vi "Read Voltage.vi"(8 "error in)":errorcluster, 11 "Voltmeter CFG in":refnum<class "Voltmeter CFG.lvclass">) -> (0 "error out":errorcluster, 2 "Voltage":dbl format="%#_g V", 3 "Voltmeter CFG out":refnum<class "Voltmeter CFG.lvclass">)   [LabVIEW 2023, in "RIGOL DS1054Z.lvlib" / "Voltmeter CFG.lvclass"]
uses:
  Voltmeter CFG.lvclass
  <vilib>/Analysis/baseanly.llb/Mean (DBL).vi
  Voltmeter CFG.lvclass/Voltmeter CFG.ctl
  <vilib>/Analysis/NI_AALBase.lvlib
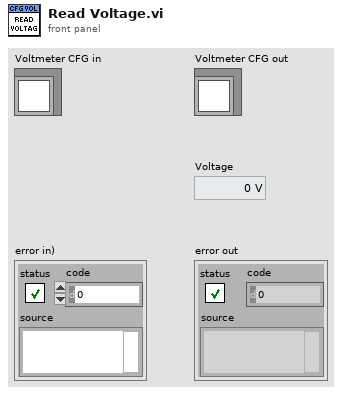
[diagram p1: front panel]
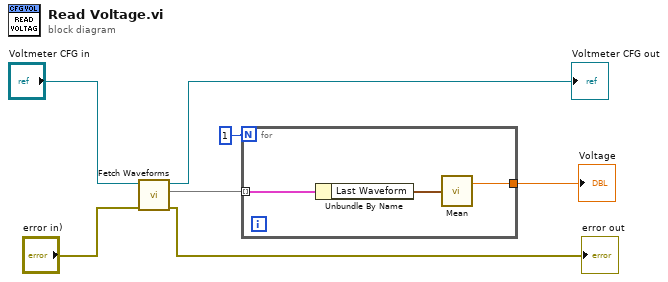
[diagram p0: block diagram]
diagram:
  n1 = call-dynamic "Fetch Waveforms.vi"("error in"="error in)", "object in"="Voltmeter CFG in") -> ("error out"=→"error out":errorcluster, "Last Waveforms"=w4:map{u8, waveform(dbl)}, "object out"=→"Voltmeter CFG out":refnum<class "Voltmeter CFG.lvclass">)  [unwired: 7 in]
  n2 = for {
    N: 1 -> [_]
    tunnel: [w10] -> w5
    tunnel: w4 -> [w9] mode=indexing
    n3 = Unbundle By Name(w9) -> ("Last Waveform"=w8:waveform(dbl))
    n4 = call-poly <vilib>:"Mean.vi"("X"=w8) -> ("mean"=w10:dbl)  [unwired: 1 out]
  }
  "Voltage" <- w5
